vi "Toggle.vi"(8 "error in (no error)":errorcluster, 11 "EpiWrapper in":refnum<class "EpiWrapper.lvclass">) -> (0 "error out":errorcluster, 3 "EpiWrapper out":refnum<class "EpiWrapper.lvclass">)   [LabVIEW 2012, in "EpiWrapper.lvclass"]
uses:
  EpiWrapper.lvclass
  Controls/Input_Lables.ctl
  EpiWrapper.lvclass/EpiWrapper.ctl
panel:
  in  "Disabled":T1(ring)=enum."Disabled and Grayed Out"
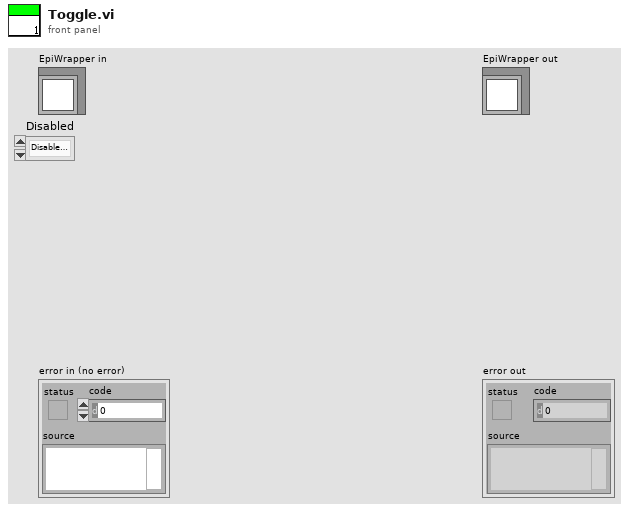
[diagram p1: front panel]
types:
  T1 = enum8{"Enabled", "Disabled", "Disabled and Grayed Out"}
  T2 = typedef "Input_Lables.ctl" = cluster{"Input_Cont[0]":string, "Input_Cont[1]":string, "Input_Cont[2]":string, "Input_Cont[3]":string, "Input_Cont[4]":string}
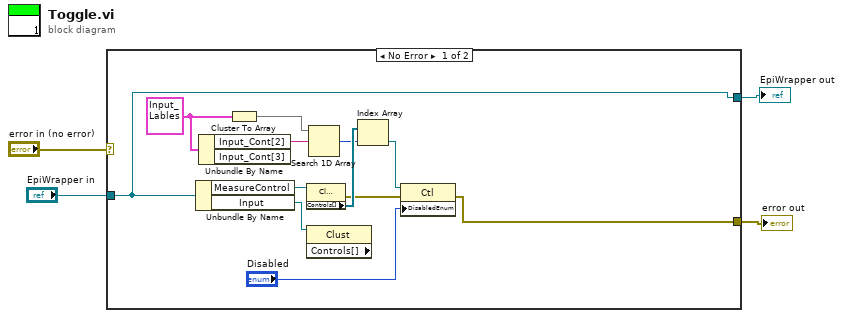
[diagram p0: block diagram]
diagram:
  n1 = case shown="No Error" "error in (no error)" {
    selector: "error in (no error)" -> [_ w18]
    tunnel: [w6 w18] -> w3
    tunnel: [w5 w17] -> w1
    tunnel: "EpiWrapper in" -> [w5 w17]
    frame No Error {
      w14 = T2 {"Input_Cont[0]"="Wafer ID", "Input_Cont[1]"="Test", "Input_Cont[2]"="New", "Input_Cont[3]"="Save", "Input_Cont[4]"="Load"} ("cluster")
      n2 = Unbundle By Name(w5) -> ("MeasureControl"=w15:refnum<vi>, "Input"=w16:refnum<vi>)
      n3 = Unbundle By Name(w14) -> ("Input_Cont[2]"=w12:string)  [unwired: 1 out]
      n4 = Cluster To Array(cluster=w14) -> (array=w13:string[])
      n5 = property class="Clust (strict)"(reference=w15) -> (error out=w7:errorcluster, "Controls[]"=w11:refnum<vi>[])  [unwired: 1 in, 1 out]
      n6 = property class="Clust" props=["Controls[]"](reference=w16) -> ()  [unwired: 1 in, 3 out]
      n7 = Search 1D Array(1D array=w13, element=w12) -> (index of element=w10:i32)  [unwired: 1 in]
      n8 = Index Array(array=w11, index=w10) -> (element=w9:refnum<vi>)
      n9 = property class="Ctl"(reference=w9, error in=w7, "DisabledEnum"="Disabled") -> (error out=w6:errorcluster)  [unwired: 1 out]
    }
    frame Error {
    }
  }
  "error out" <- w3
  "EpiWrapper out" <- w1
